vi "Main.vi"(7 "sweep rate, /min":dbl=0.2, 8 "sweep to:":dbl=-0.5, 9 "sweep":T6(radio)=enum."time_sweep") -> ()   [LabVIEW 2017] (continued)
            n4932 = property on="Continuous Sweep" class="Bool (strict)"("DisabledEnum"=w6382) -> ()  [unwired: 2 in, 2 out]
            n4933 = property on="Step and Hyerloop Setups" class="TabCtl (strict)"() -> ("Pages"=w6368:refnum<vi>[])  [unwired: 2 in, 2 out]
            n4934 = property on="Step and Hyerloop Setups" class="TabCtl (strict)"() -> ("Pages"=w6374:refnum<vi>[])  [unwired: 2 in, 2 out]
            n4935 = Index Array(array=w6377, index=2) -> (element=w6378:refnum<vi>)
            n4936 = Index Array(array=w6368, index=3) -> (element=w6367:refnum<vi>)
            n4937 = Index Array(array=w6374, index=1) -> (element=w6373:refnum<vi>)
            n4938 = property on="Continuous Sweep" class="Bool (strict)"("Value"=FALSE ("Continuous Sweep")) -> ()  [unwired: 2 in, 2 out]
            n4939 = property on="SuperHyper" class="Bool (strict)"("Value"=FALSE ("SuperHyper")) -> ()  [unwired: 2 in, 2 out]
            n4940 = property class="Page"(reference=w6378, "PageVis"=FALSE ("Page Visible")) -> ()  [unwired: 1 in, 2 out]
            n4941 = property on="MappingName" class="Str"("Visible"=TRUE) -> ()  [unwired: 2 in, 2 out]
            n4942 = property class="Page"(reference=w6367, "PageVis"=FALSE ("Page Visible")) -> ()  [unwired: 1 in, 2 out]
            n4943 = property class="Page"(reference=w6373, "PageVis"=TRUE ("Page Visible")) -> ()  [unwired: 1 in, 2 out]
            n4944 = property on="step" class="RadioBtnsControl (strict)"("DisabledEnum"=w6380) -> ()  [unwired: 2 in, 2 out]
            n4945 = property on="diagonal step" class="Bool (strict)"("DisabledEnum"=w6380) -> ()  [unwired: 2 in, 2 out]
            n4946 = property on="Step Offset" class="DigNum (strict)"("DisabledEnum"=w6380) -> ()  [unwired: 2 in, 2 out]
            n4947 = property on="Step Slope" class="DigNum (strict)"("DisabledEnum"=w6380) -> ()  [unwired: 2 in, 2 out]
            n4948 = property on="FieldRate(T/min)" class="DigNum (strict)"("DisabledEnum"=w6380) -> ()  [unwired: 2 in, 2 out]
            n4949 = property on="iPS _addr_step" class="VISAName"("DisabledEnum"=w6380) -> ()  [unwired: 2 in, 2 out]
            n4950 = property on="wait between sweeps(s)" class="DigNum (strict)"("DisabledEnum"=w6380) -> ()  [unwired: 2 in, 2 out]
            n4951 = property on="2336A_addr_step" class="VISAName"("DisabledEnum"=w6380) -> ()  [unwired: 2 in, 2 out]
            n4952 = property on="iTC_addr_step" class="VISAName"("DisabledEnum"=w6380) -> ()  [unwired: 2 in, 2 out]
            n4953 = property on="Start Mapping" class="Bool"("DisabledEnum"=w6380) -> ()  [unwired: 2 in, 2 out]
            n4954 = property on="2400_1_addr_step" class="DigNum (strict)"("DisabledEnum"=w6380) -> ()  [unwired: 2 in, 2 out]
            n4955 = property on="Tolerance_Step" class="DigNum (strict)"("DisabledEnum"=w6380) -> ()  [unwired: 2 in, 2 out]
            n4956 = property on="Wait Between Step(s)" class="DigNum (strict)"("DisabledEnum"=w6380) -> ()  [unwired: 2 in, 2 out]
            n4957 = property on="2400_2_addr_step" class="DigNum (strict)"("DisabledEnum"=w6380) -> ()  [unwired: 2 in, 2 out]
            n4958 = property on="HyperLoop" class="Bool (strict)"("DisabledEnum"=w6380) -> ()  [unwired: 2 in, 2 out]
          }
          frame False {
            w6393 = T12."Disabled and Grayed Out" ("Disabled")
            w6400 = T12."Enabled" ("Disabled")
            n4959 = property on="Ramp\n Down" class="Bool"("DisabledEnum"=w6400) -> ()  [unwired: 2 in, 2 out]
            n4960 = property on="iTC_addr_sweep" class="VISAName"("DisabledEnum"=w6400) -> ()  [unwired: 2 in, 2 out]
            n4961 = property on="sweep" class="RadioBtnsControl (strict)"("DisabledEnum"=w6400) -> ()  [unwired: 2 in, 2 out]
            n4962 = property on="2182A 1 addr" class="DigNum (strict)"("DisabledEnum"=w6400) -> ()  [unwired: 2 in, 2 out]
            n4963 = property on="2182A 2 addr" class="DigNum (strict)"("DisabledEnum"=w6400) -> ()  [unwired: 2 in, 2 out]
            n4964 = property on="2182A 3 addr" class="DigNum (strict)"("DisabledEnum"=w6400) -> ()  [unwired: 2 in, 2 out]
            n4965 = property on="2182A 4 addr" class="DigNum (strict)"("DisabledEnum"=w6400) -> ()  [unwired: 2 in, 2 out]
            n4966 = property on="2400 1 addr" class="DigNum (strict)"("DisabledEnum"=w6400) -> ()  [unwired: 2 in, 2 out]
            n4967 = property on="iPS_addr_sweep" class="VISAName"("DisabledEnum"=w6400) -> ()  [unwired: 2 in, 2 out]
            n4968 = property on="Sweep Down" class="Bool"("DisabledEnum"=w6400) -> ()  [unwired: 2 in, 2 out]
            n4969 = property on="SR830 2 addr" class="DigNum (strict)"("DisabledEnum"=w6400) -> ()  [unwired: 2 in, 2 out]
            n4970 = property on="SR830 3 addr" class="DigNum (strict)"("DisabledEnum"=w6400) -> ()  [unwired: 2 in, 2 out]
            n4971 = property on="2400 2 addr" class="DigNum (strict)"("DisabledEnum"=w6400) -> ()  [unwired: 2 in, 2 out]
            n4972 = property on="2400 3 addr" class="DigNum (strict)"("DisabledEnum"=w6400) -> ()  [unwired: 2 in, 2 out]
            n4973 = property on="2336A addr" class="VISAName"("DisabledEnum"=w6400) -> ()  [unwired: 2 in, 2 out]
            n4974 = property on="SR830 1 addr" class="DigNum (strict)"("DisabledEnum"=w6400) -> ()  [unwired: 2 in, 2 out]
            n4975 = property on="SR830 4 addr" class="DigNum (strict)"("DisabledEnum"=w6400) -> ()  [unwired: 2 in, 2 out]
            n4976 = property on="Ramp \nUp" class="Bool"("DisabledEnum"=w6400) -> ()  [unwired: 2 in, 2 out]
            n4977 = property on="Sweep Up" class="Bool"("DisabledEnum"=w6400) -> ()  [unwired: 2 in, 2 out]
            n4978 = property on="Step and Hyerloop Setups" class="TabCtl (strict)"() -> ("Pages"=w6388:refnum<vi>[])  [unwired: 2 in, 2 out]
            n4979 = property on="Step and Hyerloop Setups" class="TabCtl (strict)"() -> ("Pages"=w6387:refnum<vi>[])  [unwired: 2 in, 2 out]
            n4980 = property on="Tolerance_Sweep" class="DigNum (strict)"("DisabledEnum"=w6400) -> ()  [unwired: 2 in, 2 out]
            n4981 = property on="Continuous Sweep" class="Bool (strict)"("DisabledEnum"=w6400) -> ()  [unwired: 2 in, 2 out]
            n4982 = property on="Step and Hyerloop Setups" class="TabCtl (strict)"() -> ("Pages"=w6398:refnum<vi>[])  [unwired: 2 in, 2 out]
            n4983 = Index Array(array=w6388, index=2) -> (element=w6389:refnum<vi>)
            n4984 = Index Array(array=w6387, index=3) -> (element=w6386:refnum<vi>)
            n4985 = property on="MappingName" class="Str"("Visible"=FALSE) -> ()  [unwired: 2 in, 2 out]
            n4986 = Index Array(array=w6398, index=1) -> (element=w6397:refnum<vi>)
            n4987 = property class="Page"(reference=w6389, "PageVis"=FALSE ("Page Visible")) -> ()  [unwired: 1 in, 2 out]
            n4988 = property on="SuperHyper" class="Bool (strict)"("Value"=FALSE ("SuperHyper")) -> ()  [unwired: 2 in, 2 out]
            n4989 = property class="Page"(reference=w6386, "PageVis"=FALSE ("Page Visible")) -> ()  [unwired: 1 in, 2 out]
            n4990 = property on="HyperLoop" class="Bool (strict)"("Value"=FALSE ("HyperLoop")) -> ()  [unwired: 2 in, 2 out]
            n4991 = property class="Page"(reference=w6397, "PageVis"=FALSE ("Page Visible")) -> ()  [unwired: 1 in, 2 out]
            n4992 = property on="step" class="RadioBtnsControl (strict)"("DisabledEnum"=w6393) -> ()  [unwired: 2 in, 2 out]
            n4993 = property on="diagonal step" class="Bool (strict)"("DisabledEnum"=w6393) -> ()  [unwired: 2 in, 2 out]
            n4994 = property on="Step Offset" class="DigNum (strict)"("DisabledEnum"=w6393) -> ()  [unwired: 2 in, 2 out]
            n4995 = property on="Step Slope" class="DigNum (strict)"("DisabledEnum"=w6393) -> ()  [unwired: 2 in, 2 out]
            n4996 = property on="iPS _addr_step" class="VISAName"("DisabledEnum"=w6393) -> ()  [unwired: 2 in, 2 out]
            n4997 = property on="wait between sweeps(s)" class="DigNum (strict)"("DisabledEnum"=w6393) -> ()  [unwired: 2 in, 2 out]
            n4998 = property on="2336A_addr_step" class="VISAName"("DisabledEnum"=w6393) -> ()  [unwired: 2 in, 2 out]
            n4999 = property on="iTC_addr_step" class="VISAName"("DisabledEnum"=w6393) -> ()  [unwired: 2 in, 2 out]
            n5000 = property on="Start Mapping" class="Bool"("DisabledEnum"=w6393) -> ()  [unwired: 2 in, 2 out]
            n5001 = property on="2400_1_addr_step" class="DigNum (strict)"("DisabledEnum"=w6393) -> ()  [unwired: 2 in, 2 out]
            n5002 = property on="Wait Between Step(s)" class="DigNum (strict)"("DisabledEnum"=w6393) -> ()  [unwired: 2 in, 2 out]
            n5003 = property on="2400_2_addr_step" class="DigNum (strict)"("DisabledEnum"=w6393) -> ()  [unwired: 2 in, 2 out]
            n5004 = property on="FieldRate(T/min)" class="DigNum (strict)"("DisabledEnum"=w6393) -> ()  [unwired: 2 in, 2 out]
            n5005 = property on="Tolerance_Step" class="DigNum (strict)"("DisabledEnum"=w6393) -> ()  [unwired: 2 in, 2 out]
            n5006 = property on="HyperLoop" class="Bool (strict)"("DisabledEnum"=w6393) -> ()  [unwired: 2 in, 2 out]
          }
        }
      }
      event "Change Sweep Range": Value Change {
        n5007 = event-data() -> ()  [unwired: 1 in, 6 out]
        n5008 = property on="Change Sweep Range" class="Bool (strict)"() -> ("Value"=w6401:bool)  [unwired: 2 in, 2 out]
        n5009 = case shown="False" w6401 {
          frame False {
            w6402 = FALSE ("Visible")
            n5010 = property on="UpLimitValue" class="DigNum (strict)"("Visible"=w6402) -> ()  [unwired: 2 in, 2 out]
            n5011 = property on="DownLimitValue" class="DigNum (strict)"("Visible"=w6402) -> ()  [unwired: 2 in, 2 out]
            n5012 = property on="Generate" class="Bool"("Visible"=w6402) -> ()  [unwired: 2 in, 2 out]
            n5013 = property on="Offset_Up" class="DigNum (strict)"("Visible"=w6402) -> ()  [unwired: 2 in, 2 out]
            n5014 = property on="Down          Up" class="Tbl (strict)"("Visible"=w6402) -> ()  [unwired: 2 in, 2 out]
            n5015 = property on="Slope" class="DigNum (strict)"("Visible"=w6402) -> ()  [unwired: 2 in, 2 out]
            n5016 = property on="Offset_Down" class="DigNum (strict)"("Visible"=w6402) -> ()  [unwired: 2 in, 2 out]
          }
          frame True {
            w6403 = TRUE ("Visible")
            n5017 = property on="UpLimitValue" class="DigNum (strict)"("Visible"=w6403) -> ()  [unwired: 2 in, 2 out]
            n5018 = property on="Generate" class="Bool"("Visible"=w6403) -> ()  [unwired: 2 in, 2 out]
            n5019 = property on="DownLimitValue" class="DigNum (strict)"("Visible"=w6403) -> ()  [unwired: 2 in, 2 out]
            n5020 = property on="Offset_Up" class="DigNum (strict)"("Visible"=w6403) -> ()  [unwired: 2 in, 2 out]
            n5021 = property on="Down          Up" class="Tbl (strict)"("Visible"=w6403) -> ()  [unwired: 2 in, 2 out]
            n5022 = property on="Slope" class="DigNum (strict)"("Visible"=w6403) -> ()  [unwired: 2 in, 2 out]
            n5023 = property on="Offset_Down" class="DigNum (strict)"("Visible"=w6403) -> ()  [unwired: 2 in, 2 out]
          }
        }
      }
      event "Generate": Value Change {
        n5024 = event-data() -> ()  [unwired: 1 in, 6 out]
        n5025 = stacked-sequence {
          frame #0 {
            # "Initialize the background colours of cells"
            n5026 = property on="Down          Up" class="Tbl (strict)"("Active Cell"=cluster{"Row":i32, "Column":i32} {"Row"=-2, "Column"=-2}, "Cell BG Color"=u32 16448250 ("Active Cell:Cell Background Color")) -> ()  [unwired: 2 in, 2 out]
          }
          frame #1 {
            # "Fill the tables"
            n5027 = property on="Step values" class="Tbl (strict)"() -> ("Value"=w6413:string[][])  [unwired: 2 in, 2 out]
            n5028 = Index Array(array=w6413, index (col)=0 ("index (row)")) -> (element=w6410:string[])  [unwired: 1 in]
            n5029 = Array Size(array=w6410) -> (size(s)=w6412:i32)
            n5030 = for {
              N: w6412 -> [_]
              tunnel: [w6433] -> w6409 mode=indexing
              tunnel: [w6432] -> w6408 mode=indexing
              i -> [w6429]
              n5031 = property on="Step values" class="Tbl (strict)"() -> ("Value"=w6431:string[][])  [unwired: 2 in, 2 out]
              n5032 = property on="Slope" class="DigNum (strict)"() -> ("Value"=w6435:dbl)  [unwired: 2 in, 2 out]
              n5033 = Index Array(array=w6431, index (row)=w6429, index (col)=0 ("disabled index (col)")) -> (element=w6428:string)
              n5034 = Fract/Exp String To Number(string=w6428) -> (number=w6414:dbl)  [unwired: 3 in, 1 out]
              n5035 = property on="Offset_Up" class="DigNum (strict)"() -> ("Value"=w6434:dbl)  [unwired: 2 in, 2 out]
              n5036 = Multiply(x=w6414, y=w6435) -> (x*y=w6425:dbl)
              n5037 = property on="Offset_Down" class="DigNum (strict)"() -> ("Value"=w6426:dbl)  [unwired: 2 in, 2 out]
              n5038 = property on="UpLimitValue" class="DigNum (strict)"() -> ("Value"=w6420:dbl)  [unwired: 2 in, 2 out]
              n5039 = Add(x=w6425, y=w6434) -> (x+y=w6421:dbl)
              n5040 = Add(x=w6426, y=w6425) -> (x+y=w6424:dbl)
              n5041 = property on="DownLimitValue" class="DigNum (strict)"() -> ("Value"=w6423:dbl)  [unwired: 2 in, 2 out]
              n5042 = property on="Change Doule Sweep OffSet" class="Bool (strict)"() -> ("Value"=w6419:bool)  [unwired: 2 in, 2 out]
              n5043 = Less?(x=w6421, y=w6420) -> (x < y?=w6422:bool)
              n5044 = Greater?(x=w6424, y=w6423) -> (0:w6427:bool)
              n5045 = Select(t=w6421, s=w6422, f=w6420) -> (s? t:f=w6416:dbl)
              n5046 = Select(t=w6424, s=w6427, f=w6423) -> (s? t:f=w6417:dbl)
              n5047 = case shown="True" w6419 {
                tunnel: [w6437 w6449] -> w6418
                tunnel: w6417 -> [w6437 w6445]
                tunnel: [w6436 w6448] -> w6415
                tunnel: w6416 -> [w6436 w6441]
                tunnel: w6414 -> [_ w6453]
                frame False {
                }
                frame True {
                  n5048 = property on="Slope" class="DigNum (strict)"() -> ("Value"=w6446:dbl)  [unwired: 2 in, 2 out]
                  n5049 = property on="SlaveUpLimit" class="DigNum (strict)"() -> ("Value"=w6454:dbl)  [unwired: 2 in, 2 out]
                  n5050 = property on="SlaveDownLimit" class="DigNum (strict)"() -> ("Value"=w6455:dbl)  [unwired: 2 in, 2 out]
                  n5051 = Absolute Value(x=w6441) -> (abs(x)=w6440:dbl)
                  n5052 = Subtract(x=w6454, y=w6453) -> (x-y=w6451:dbl)
                  n5053 = Subtract(x=w6455, y=w6453) -> (x-y=w6452:dbl)
                  n5054 = Absolute Value(x=w6445) -> (abs(x)=w6444:dbl)
                  n5055 = Divide(x=w6452, y=w6446) -> (x/y=w6443:dbl)
                  n5056 = Divide(x=w6451, y=w6446) -> (x/y=w6438:dbl)
                  n5057 = Absolute Value(x=w6438) -> (abs(x)=w6439:dbl)
                  n5058 = Absolute Value(x=w6443) -> (abs(x)=w6442:dbl)
                  n5059 = Less?(x=w6442, y=w6444) -> (x < y?=w6450:bool)
                  n5060 = Less?(x=w6439, y=w6440) -> (x < y?=w6447:bool)
                  n5061 = Select(t=w6438, s=w6447, f=w6441) -> (s? t:f=w6448:dbl)
                  n5062 = Select(t=w6443, s=w6450, f=w6445) -> (s? t:f=w6449:dbl)
                }
              }
              n5063 = Number To Fractional String(number=w6415) -> (F-format string=w6432:string)  [unwired: 3 in]
              n5064 = Number To Fractional String(number=w6418) -> (F-format string=w6433:string)  [unwired: 3 in]
            }
            n5065 = Build Array(w6409, w6408) -> (w6407:string[][])
            n5066 = Transpose 2D Array(2D array=w6407) -> (transposed array=w6406:string[][])
            n5067 = property on="Down          Up" class="Tbl (strict)"("Value"=w6406) -> ()  [unwired: 2 in, 2 out]
          }
        }
      }
      event "HyperLoop": Value Change {
        n5068 = event-data() -> ()  [unwired: 1 in, 6 out]
        n5069 = property on="HyperLoop" class="Bool (strict)"() -> ("Value"=w6456:bool)  [unwired: 2 in, 2 out]
        n5070 = case shown="True" w6456 {
          frame False {
            n5071 = property on="Step and Hyerloop Setups" class="TabCtl (strict)"() -> ("Pages"=w6462:refnum<vi>[])  [unwired: 2 in, 2 out]
            n5072 = Index Array(array=w6462, index=3) -> (element=w6461:refnum<vi>)
            n5073 = property on="SuperHyper" class="Bool (strict)"("Value"=FALSE ("SuperHyper")) -> ()  [unwired: 2 in, 2 out]
            n5074 = property on="HyperLoop" class="Bool (strict)"("Value"=FALSE ("HyperLoop")) -> ()  [unwired: 2 in, 2 out]
            n5075 = property class="Page"(reference=w6461, "PageVis"=FALSE ("Page Visible")) -> ()  [unwired: 1 in, 2 out]
            n5076 = property on="Step and Hyerloop Setups" class="TabCtl (strict)"() -> ("Pages"=w6467:refnum<vi>[])  [unwired: 2 in, 2 out]
            n5077 = Index Array(array=w6467, index=2) -> (element=w6466:refnum<vi>)
            n5078 = property on="Start Mapping" class="Bool"("DisabledEnum"=T12."Enabled" ("Disabled")) -> ()  [unwired: 2 in, 2 out]
            n5079 = property class="Page"(reference=w6466, "PageVis"=FALSE ("Page Visible")) -> ()  [unwired: 1 in, 2 out]
          }
          frame True {
            n5080 = property on="Step and Hyerloop Setups" class="TabCtl (strict)"() -> ("Pages"=w6473:refnum<vi>[])  [unwired: 2 in, 2 out]
            n5081 = Index Array(array=w6473, index=2) -> (element=w6471:refnum<vi>)
            n5082 = property on="Start Mapping" class="Bool"("DisabledEnum"=T12."Disabled and Grayed Out" ("Disabled")) -> ()  [unwired: 2 in, 2 out]
            n5083 = property class="Page"(reference=w6471, "PageVis"=TRUE ("Page Visible")) -> ()  [unwired: 1 in, 2 out]
            n5084 = property on="SuperHyper" class="Bool (strict)"("Value"=FALSE ("SuperHyper")) -> ()  [unwired: 2 in, 2 out]
          }
        }
      }
      event "SuperHyper": Value Change {
        n5085 = event-data() -> ()  [unwired: 1 in, 6 out]
        n5086 = property on="SuperHyper" class="Bool (strict)"() -> ("Value"=w6474:bool)  [unwired: 2 in, 2 out]
        n5087 = case shown="True" w6474 {
          frame False {
            n5088 = property on="Step and Hyerloop Setups" class="TabCtl (strict)"() -> ("Pages"=w6479:refnum<vi>[])  [unwired: 2 in, 2 out]
            n5089 = Index Array(array=w6479, index=3) -> (element=w6478:refnum<vi>)
            n5090 = property on="Start HyperLoop" class="Bool"("DisabledEnum"=T12."Enabled" ("Disabled")) -> ()  [unwired: 2 in, 2 out]
            n5091 = property class="Page"(reference=w6478, "PageVis"=FALSE ("Page Visible")) -> ()  [unwired: 1 in, 2 out]
          }
          frame True {
            n5092 = property on="Step  Setups" class="TabCtl (strict)"() -> ("Pages"=w6484:refnum<vi>[])  [unwired: 2 in, 2 out]
            n5093 = Index Array(array=w6484, index=3) -> (element=w6482:refnum<vi>)
            n5094 = property class="Page"(reference=w6482, "PageVis"=TRUE ("Page Visible")) -> ()  [unwired: 1 in, 2 out]
            n5095 = property on="Start HyperLoop" class="Bool"("DisabledEnum"=T12."Disabled and Grayed Out" ("Disabled")) -> ()  [unwired: 2 in, 2 out]
          }
        }
      }
      event "Quit": Value Change {
        n5096 = event-data() -> ()  [unwired: 1 in, 6 out]
        n5097 = Flush Queue(queue=w6487) -> (queue out=w6486:refnum<queue>)  [unwired: 1 in, 2 out]
        n5098 = Enqueue Element(queue=w6486, element="Quit") -> ()  [unwired: 2 in, 3 out]
      }
      event "Populate step table?": Value Change {
        n5099 = event-data() -> ()  [unwired: 1 in, 6 out]
        n5100 = stacked-sequence {
          frame #0 {
            # "Initialize the background colours of cells"
            n5101 = property on="Step values" class="Tbl (strict)"("Active Cell"=cluster{"Row":i32, "Column":i32} {"Row"=-2, "Column"=-2}, "Cell BG Color"=u32 16448250 ("Active Cell:Cell Background Color")) -> ()  [unwired: 2 in, 2 out]
          }
          frame #1 {
            # "Fill the tables"
            n5102 = property on="to" class="DigNum (strict)"() -> ("Value"=w6492:dbl)  [unwired: 2 in, 2 out]
            n5103 = property on="step" class="DigNum (strict)"() -> ("Value"=w6491:dbl)  [unwired: 2 in, 2 out]
            n5104 = property on="from" class="DigNum (strict)"() -> ("Value"=w6493:dbl)  [unwired: 2 in, 2 out]
            n5105 = Subtract(x=w6493, y=w6492) -> (x-y=w6500:dbl)
            n5106 = Divide(x=w6500, y=w6491) -> (x/y=w6499:dbl)
            n5107 = Sign(1:w6500) -> (0:w6503:dbl)
            n5108 = Absolute Value(x=w6499) -> (abs(x)=w6498:dbl)
            n5109 = Negate(x=w6503) -> (-x=w6495:dbl)
            n5110 = Round Toward -Infinity(1:w6498) -> (0:w6497:dbl)
            n5111 = Increment(x=w6497) -> (x+1=w6496:dbl)
            n5112 = for {
              N: w6496 -> [_]
              tunnel: w6493 -> [w6509]
              tunnel: w6495 -> [w6510]
              tunnel: w6491 -> [w6512]
              tunnel: [w6506] -> w6501 mode=indexing
              i -> [w6504]
              n5113 = Multiply(x=w6512, y=w6504) -> (x*y=w6511:dbl)
              n5114 = Multiply(x=w6510, y=w6511) -> (x*y=w6508:dbl)
              n5115 = Add(x=w6509, y=w6508) -> (x+y=w6507:dbl)
              n5116 = Number To Fractional String(number=w6507, precision (6)=i16 6) -> (F-format string=w6506:string)  [unwired: 2 in]
            }
            n5117 = Build Array(w6501) -> (w6502:string[][])
            n5118 = Transpose 2D Array(2D array=w6502) -> (transposed array=w6494:string[][])
            n5119 = property on="Step values" class="Tbl (strict)"("Value"=w6494) -> ()  [unwired: 2 in, 2 out]
          }
          frame #2 {
            # "Calculate the measurement time and estimate the finished time"
            n5120 = property on="upper limit" class="DigNum (strict)"() -> ("Value"=w6544:dbl)  [unwired: 2 in, 2 out]
            n5121 = property on="lower limit" class="DigNum (strict)"() -> ("Value"=w6545:dbl)  [unwired: 2 in, 2 out]
            n5122 = Subtract(x=w6545, y=w6544) -> (x-y=w6543:dbl)
            n5123 = property on="Down Rate" class="DigNum (strict)"() -> ("Value"=w6540:dbl)  [unwired: 2 in, 2 out]
            n5124 = property on="Up Rate" class="DigNum (strict)"() -> ("Value"=w6542:dbl)  [unwired: 2 in, 2 out]
            n5125 = Absolute Value(x=w6543) -> (abs(x)=w6541:dbl)
            n5126 = property on="step" class="RadioBtnsControl (strict)"() -> ("Value"=w6520:T8)  [unwired: 2 in, 2 out]
            n5127 = Divide(x=w6541, y=w6542) -> (x/y=w6539:dbl)
            n5128 = Divide(x=w6541, y=w6540) -> (x/y=w6538:dbl)
            n5129 = case shown="\"iPS_step\"" w6520 {
              tunnel: [w6546 0.0] -> w6516
              frame "iPS_step" {
                n5130 = property on="step" class="DigNum (strict)"() -> ("Value"=w6550:dbl)  [unwired: 2 in, 2 out]
                n5131 = property on="FieldRate(T/min)" class="DigNum (strict)"() -> ("Value"=w6549:dbl)  [unwired: 2 in, 2 out]
                n5132 = Divide(x=w6550, y=w6549) -> (x/y=w6548:dbl)
                n5133 = Multiply(x=w6548, y=60.0) -> (x*y=w6546:dbl)
              }
              frame "V2400_1_Step".."iTC_step", Default {
              }
            }
            n5134 = property on="Wait Between Step(s)" class="DigNum (strict)"() -> ("Value"=w6535:i32)  [unwired: 2 in, 2 out]
            n5135 = Add(x=w6539, y=w6538) -> (x+y=w6537:dbl)
            n5136 = Multiply(x=w6537, y=60.0) -> (x*y=w6536:dbl)
            n5137 = property on="Step values" class="Tbl (strict)"() -> ("Value"=w6530:string[][])  [unwired: 2 in, 2 out]
            n5138 = property on="wait between sweeps(s)" class="DigNum (strict)"() -> ("Value"=w6533:u32)  [unwired: 2 in, 2 out]
            n5139 = Add(x=w6536, y=w6535) -> (x+y=w6534:dbl)
            n5140 = Array Size(array=w6530) -> (size(s)=w6529:i32[])
            n5141 = Index Array(array=w6529, index=0) -> (element=w6515:i32)
            n5142 = Add(x=w6534, y=w6533) -> (x+y=w6519:dbl)
            n5143 = Multiply(x=w6515, y=w6519) -> (x*y=w6517:dbl)
            n5144 = Decrement(x=w6515) -> (x-1=w6514:i32)
            n5145 = Multiply(x=w6514, y=w6516) -> (x*y=w6513:dbl)
            n5146 = Add(x=w6517, y=w6513) -> (x+y=w6518:dbl)
            n5147 = Get Date/Time In Seconds() -> (seconds since 1Jan1904=w6532:timestamp)
            n5148 = Add(x=w6518, y=w6532) -> (x+y=w6528:timestamp)
            n5149 = Quotient & Remainder(x=w6518, y=3600.0) -> (x-y*floor(x/y)=w6531:dbl, floor(x/y)=w6527:dbl)
            n5150 = Quotient & Remainder(x=w6531, y=60.0) -> (x-y*floor(x/y)=w6525:dbl, floor(x/y)=w6526:dbl)
            n5151 = property on="SS:" class="DigNum (strict)"("Value"=w6525) -> ()  [unwired: 2 in, 2 out]
            n5152 = property on="MM:" class="DigNum (strict)"("Value"=w6526) -> ()  [unwired: 2 in, 2 out]
            n5153 = property on="HH:" class="DigNum (strict)"("Value"=w6527) -> ()  [unwired: 2 in, 2 out]
            n5154 = property on="Finish Time" class="AbsTime (strict)"("Value"=w6528) -> ()  [unwired: 2 in, 2 out]
          }
        }
      }
      event "Hidden_HyperLoop_Swap": Value Change {
        n5155 = event-data() -> ()  [unwired: 1 in, 6 out]
        n5156 = stacked-sequence {
          frame #0 {
            # "Initialize the background colours of cells"
            n5157 = property on="Step values" class="Tbl (strict)"("Active Cell"=cluster{"Row":i32, "Column":i32} {"Row"=-2, "Column"=-2}, "Cell BG Color"=u32 16448250 ("Active Cell:Cell Background Color")) -> ()  [unwired: 2 in, 2 out]
          }
          frame #1 {
            # "Fill the tables"
            n5158 = property on="Step values" class="Tbl (strict)"() -> ("Value"=w6559:string[][])  [unwired: 2 in, 2 out]
            n5159 = Index Array(array=w6559, index (col)=0 ("disabled index (col)")) -> (element=w6557:string[])  [unwired: 1 in]
            n5160 = Reverse 1D Array(array=w6557) -> (reversed array=w6556:string[])
            n5161 = Build Array(w6556) -> (w6555:string[][])
            n5162 = Transpose 2D Array(2D array=w6555) -> (transposed array=w6554:string[][])
            n5163 = property on="Step values" class="Tbl (strict)"("Value"=w6554) -> ()  [unwired: 2 in, 2 out]
          }
          frame #2 {
            # "Calculate the measurement time and estimate the finished time"
            n5164 = property on="upper limit" class="DigNum (strict)"() -> ("Value"=w6591:dbl)  [unwired: 2 in, 2 out]
            n5165 = property on="lower limit" class="DigNum (strict)"() -> ("Value"=w6592:dbl)  [unwired: 2 in, 2 out]
            n5166 = Subtract(x=w6592, y=w6591) -> (x-y=w6590:dbl)
            n5167 = property on="Down Rate" class="DigNum (strict)"() -> ("Value"=w6587:dbl)  [unwired: 2 in, 2 out]
            n5168 = property on="Up Rate" class="DigNum (strict)"() -> ("Value"=w6589:dbl)  [unwired: 2 in, 2 out]
            n5169 = Absolute Value(x=w6590) -> (abs(x)=w6588:dbl)
            n5170 = property on="step" class="RadioBtnsControl (strict)"() -> ("Value"=w6567:T8)  [unwired: 2 in, 2 out]
            n5171 = Divide(x=w6588, y=w6589) -> (x/y=w6586:dbl)
            n5172 = Divide(x=w6588, y=w6587) -> (x/y=w6585:dbl)
            n5173 = case shown="\"iPS_step\"" w6567 {
              tunnel: [w6593 0.0] -> w6563
              frame "iPS_step" {
                n5174 = property on="step" class="DigNum (strict)"() -> ("Value"=w6597:dbl)  [unwired: 2 in, 2 out]
                n5175 = property on="FieldRate(T/min)" class="DigNum (strict)"() -> ("Value"=w6596:dbl)  [unwired: 2 in, 2 out]
                n5176 = Divide(x=w6597, y=w6596) -> (x/y=w6595:dbl)
                n5177 = Multiply(x=w6595, y=60.0) -> (x*y=w6593:dbl)
              }
              frame "V2400_1_Step".."iTC_step", Default {
              }
            }
            n5178 = property on="Wait Between Step(s)" class="DigNum (strict)"() -> ("Value"=w6582:i32)  [unwired: 2 in, 2 out]
            n5179 = Add(x=w6586, y=w6585) -> (x+y=w6584:dbl)
            n5180 = Multiply(x=w6584, y=60.0) -> (x*y=w6583:dbl)
            n5181 = property on="Step values" class="Tbl (strict)"() -> ("Value"=w6577:string[][])  [unwired: 2 in, 2 out]
            n5182 = property on="wait between sweeps(s)" class="DigNum (strict)"() -> ("Value"=w6580:u32)  [unwired: 2 in, 2 out]
            n5183 = Add(x=w6583, y=w6582) -> (x+y=w6581:dbl)
            n5184 = Array Size(array=w6577) -> (size(s)=w6576:i32[])
            n5185 = Index Array(array=w6576, index=0) -> (element=w6562:i32)
            n5186 = Add(x=w6581, y=w6580) -> (x+y=w6566:dbl)
            n5187 = Multiply(x=w6562, y=w6566) -> (x*y=w6564:dbl)
            n5188 = Decrement(x=w6562) -> (x-1=w6561:i32)
            n5189 = Multiply(x=w6561, y=w6563) -> (x*y=w6560:dbl)
            n5190 = Add(x=w6564, y=w6560) -> (x+y=w6565:dbl)
            n5191 = Get Date/Time In Seconds() -> (seconds since 1Jan1904=w6579:timestamp)
            n5192 = Add(x=w6565, y=w6579) -> (x+y=w6575:timestamp)
            n5193 = Quotient & Remainder(x=w6565, y=3600.0) -> (x-y*floor(x/y)=w6578:dbl, floor(x/y)=w6574:dbl)
            n5194 = Quotient & Remainder(x=w6578, y=60.0) -> (x-y*floor(x/y)=w6572:dbl, floor(x/y)=w6573:dbl)
            n5195 = property on="SS:" class="DigNum (strict)"("Value"=w6572) -> ()  [unwired: 2 in, 2 out]
            n5196 = property on="MM:" class="DigNum (strict)"("Value"=w6573) -> ()  [unwired: 2 in, 2 out]
            n5197 = property on="HH:" class="DigNum (strict)"("Value"=w6574) -> ()  [unwired: 2 in, 2 out]
            n5198 = property on="Finish Time" class="AbsTime (strict)"("Value"=w6575) -> ()  [unwired: 2 in, 2 out]
          }
        }
      }
      event "Populate HyperLoop table?": Value Change {
        n5199 = event-data() -> ()  [unwired: 1 in, 6 out]
        n5200 = stacked-sequence {
          frame #0 {
            n5201 = property on="HyperLoop Steps" class="Tbl (strict)"("Active Cell"=cluster{"Row":i32, "Column":i32} {"Row"=-2, "Column"=-2}, "Cell BG Color"=u32 16448250 ("Active Cell:Cell Background Color")) -> ()  [unwired: 2 in, 2 out]
          }
          frame #1 {
            n5202 = property on="to" class="DigNum (strict)"() -> ("Value"=w6603:dbl)  [unwired: 2 in, 2 out]
            n5203 = property on="step" class="DigNum (strict)"() -> ("Value"=w6602:dbl)  [unwired: 2 in, 2 out]
            n5204 = property on="from" class="DigNum (strict)"() -> ("Value"=w6604:dbl)  [unwired: 2 in, 2 out]
            n5205 = Subtract(x=w6604, y=w6603) -> (x-y=w6610:dbl)
            n5206 = Divide(x=w6610, y=w6602) -> (x/y=w6609:dbl)
            n5207 = Sign(1:w6610) -> (0:w6613:dbl)
            n5208 = Absolute Value(x=w6609) -> (abs(x)=w6608:dbl)
            n5209 = Negate(x=w6613) -> (-x=w6605:dbl)
            n5210 = Round Toward -Infinity(1:w6608) -> (0:w6607:dbl)
            n5211 = Increment(x=w6607) -> (x+1=w6606:dbl)
            n5212 = for {
              N: w6606 -> [_]
              tunnel: w6604 -> [w6619]
              tunnel: w6605 -> [w6620]
              tunnel: w6602 -> [w6622]
              tunnel: [w6616] -> w6611 mode=indexing
              i -> [w6614]
              n5213 = Multiply(x=w6622, y=w6614) -> (x*y=w6621:dbl)
              n5214 = Multiply(x=w6620, y=w6621) -> (x*y=w6618:dbl)
              n5215 = Add(x=w6619, y=w6618) -> (x+y=w6617:dbl)
              n5216 = Number To Fractional String(number=w6617, precision (6)=i16 6) -> (F-format string=w6616:string)  [unwired: 2 in]
            }
            n5217 = Build Array(w6611) -> (w6612:string[][])
            n5218 = Transpose 2D Array(2D array=w6612) -> (transposed array=w6601:string[][])
            n5219 = property on="HyperLoop Steps" class="Tbl (strict)"("Value"=w6601) -> ()  [unwired: 2 in, 2 out]
          }
          frame #2 {
            n5220 = property on="upper limit" class="DigNum (strict)"() -> ("Value"=w6657:dbl)  [unwired: 2 in, 2 out]
            n5221 = property on="lower limit" class="DigNum (strict)"() -> ("Value"=w6658:dbl)  [unwired: 2 in, 2 out]
            n5222 = Subtract(x=w6658, y=w6657) -> (x-y=w6656:dbl)
            n5223 = property on="Down Rate" class="DigNum (strict)"() -> ("Value"=w6653:dbl)  [unwired: 2 in, 2 out]
            n5224 = property on="Up Rate" class="DigNum (strict)"() -> ("Value"=w6655:dbl)  [unwired: 2 in, 2 out]
            n5225 = Absolute Value(x=w6656) -> (abs(x)=w6654:dbl)
            n5226 = property on="step" class="RadioBtnsControl (strict)"() -> ("Value"=w6634:T8)  [unwired: 2 in, 2 out]
            n5227 = Divide(x=w6654, y=w6655) -> (x/y=w6652:dbl)
            n5228 = Divide(x=w6654, y=w6653) -> (x/y=w6651:dbl)
            n5229 = case shown="\"V2400_1_Step\"..\"iTC_step\", Default" w6634 {
              tunnel: [w6659 0.0] -> w6633
              frame "iPS_step" {
                n5230 = property on="step" class="DigNum (strict)"() -> ("Value"=w6663:dbl)  [unwired: 2 in, 2 out]
                n5231 = property on="FieldRate(T/min)" class="DigNum (strict)"() -> ("Value"=w6662:dbl)  [unwired: 2 in, 2 out]
                n5232 = Divide(x=w6663, y=w6662) -> (x/y=w6661:dbl)
                n5233 = Multiply(x=w6661, y=60.0) -> (x*y=w6659:dbl)
              }
              frame "V2400_1_Step".."iTC_step", Default {
              }
            }
            n5234 = property on="Wait Between Step(s)" class="DigNum (strict)"() -> ("Value"=w6648:i32)  [unwired: 2 in, 2 out]
            n5235 = Add(x=w6652, y=w6651) -> (x+y=w6650:dbl)
            n5236 = Multiply(x=w6650, y=60.0) -> (x*y=w6649:dbl)
            n5237 = property on="HyperLoop Steps" class="Tbl (strict)"() -> ("Value"=w6629:string[][])  [unwired: 2 in, 2 out]
            n5238 = property on="wait between sweeps(s)" class="DigNum (strict)"() -> ("Value"=w6646:u32)  [unwired: 2 in, 2 out]
            n5239 = Add(x=w6649, y=w6648) -> (x+y=w6647:dbl)
            n5240 = property on="Step values" class="Tbl (strict)"() -> ("Value"=w6643:string[][])  [unwired: 2 in, 2 out]
            n5241 = Array Size(array=w6629) -> (size(s)=w6631:i32[])
            n5242 = Array Size(array=w6643) -> (size(s)=w6642:i32[])
            n5243 = Add(x=w6647, y=w6646) -> (x+y=w6636:dbl)
            n5244 = Index Array(array=w6631, index=0) -> (element=w6632:i32)
            n5245 = Index Array(array=w6642, index=0) -> (element=w6641:i32)
            n5246 = Add(x=w6636, y=w6633) -> (x+y=w6635:dbl)
            n5247 = Multiply(x=w6641, y=w6635) -> (x*y=w6628:dbl)
            n5248 = Multiply(x=w6632, y=w6628) -> (x*y=w6627:dbl)
            n5249 = Get Date/Time In Seconds() -> (seconds since 1Jan1904=w6645:timestamp)
            n5250 = Add(x=w6627, y=w6645) -> (x+y=w6623:timestamp)
            n5251 = Quotient & Remainder(x=w6627, y=3600.0) -> (x-y*floor(x/y)=w6644:dbl, floor(x/y)=w6624:dbl)
            n5252 = Quotient & Remainder(x=w6644, y=60.0) -> (x-y*floor(x/y)=w6626:dbl, floor(x/y)=w6625:dbl)
            n5253 = property on="Finish Time 2" class="AbsTime (strict)"("Value"=w6623) -> ()  [unwired: 2 in, 2 out]
            n5254 = property on="HH:" class="DigNum (strict)"("Value"=w6624) -> ()  [unwired: 2 in, 2 out]
            n5255 = property on="MM:" class="DigNum (strict)"("Value"=w6625) -> ()  [unwired: 2 in, 2 out]
            n5256 = property on="SS:" class="DigNum (strict)"("Value"=w6626) -> ()  [unwired: 2 in, 2 out]
          }
        }
      }
      event "Populate SuperHyper table?": Value Change {
        n5257 = event-data() -> ()  [unwired: 1 in, 6 out]
        n5258 = stacked-sequence {
          frame #0 {
            n5259 = property on="SuperHyper Steps" class="Tbl (strict)"("Active Cell"=cluster{"Row":i32, "Column":i32} {"Row"=-2, "Column"=-2}, "Cell BG Color"=u32 16448250 ("Active Cell:Cell Background Color")) -> ()  [unwired: 2 in, 2 out]
          }
          frame #1 {
            n5260 = property on="to" class="DigNum (strict)"() -> ("Value"=w6669:dbl)  [unwired: 2 in, 2 out]
            n5261 = property on="from" class="DigNum (strict)"() -> ("Value"=w6670:dbl)  [unwired: 2 in, 2 out]
            n5262 = property on="step" class="DigNum (strict)"() -> ("Value"=w6668:dbl)  [unwired: 2 in, 2 out]
            n5263 = Subtract(x=w6670, y=w6669) -> (x-y=w6676:dbl)
            n5264 = Divide(x=w6676, y=w6668) -> (x/y=w6675:dbl)
            n5265 = Sign(1:w6676) -> (0:w6679:dbl)
            n5266 = Absolute Value(x=w6675) -> (abs(x)=w6674:dbl)
            n5267 = Negate(x=w6679) -> (-x=w6671:dbl)
            n5268 = Round Toward -Infinity(1:w6674) -> (0:w6673:dbl)
            n5269 = Increment(x=w6673) -> (x+1=w6672:dbl)
            n5270 = for {
              N: w6672 -> [_]
              tunnel: w6670 -> [w6685]
              tunnel: w6671 -> [w6686]
              tunnel: w6668 -> [w6688]
              tunnel: [w6682] -> w6677 mode=indexing
              i -> [w6680]
              n5271 = Multiply(x=w6688, y=w6680) -> (x*y=w6687:dbl)
              n5272 = Multiply(x=w6686, y=w6687) -> (x*y=w6684:dbl)
              n5273 = Add(x=w6685, y=w6684) -> (x+y=w6683:dbl)
              n5274 = Number To Fractional String(number=w6683, precision (6)=i16 6) -> (F-format string=w6682:string)  [unwired: 2 in]
            }
            n5275 = Build Array(w6677) -> (w6678:string[][])
            n5276 = Transpose 2D Array(2D array=w6678) -> (transposed array=w6667:string[][])
            n5277 = property on="SuperHyper Steps" class="Tbl (strict)"("Value"=w6667) -> ()  [unwired: 2 in, 2 out]
          }
          frame #2 {
            n5278 = property on="upper limit" class="DigNum (strict)"() -> ("Value"=w6728:dbl)  [unwired: 2 in, 2 out]
            n5279 = property on="lower limit" class="DigNum (strict)"() -> ("Value"=w6729:dbl)  [unwired: 2 in, 2 out]
            n5280 = Subtract(x=w6729, y=w6728) -> (x-y=w6727:dbl)
            n5281 = property on="Down Rate" class="DigNum (strict)"() -> ("Value"=w6724:dbl)  [unwired: 2 in, 2 out]
            n5282 = property on="Up Rate" class="DigNum (strict)"() -> ("Value"=w6726:dbl)  [unwired: 2 in, 2 out]
            n5283 = Absolute Value(x=w6727) -> (abs(x)=w6725:dbl)
            n5284 = property on="step" class="RadioBtnsControl (strict)"() -> ("Value"=w6705:T8)  [unwired: 2 in, 2 out]
            n5285 = Divide(x=w6725, y=w6726) -> (x/y=w6723:dbl)
            n5286 = Divide(x=w6725, y=w6724) -> (x/y=w6722:dbl)
            n5287 = case shown="\"iPS_step\"" w6705 {
              tunnel: [w6730 0.0] -> w6704
              frame "iPS_step" {
                n5288 = property on="step" class="DigNum (strict)"() -> ("Value"=w6734:dbl)  [unwired: 2 in, 2 out]
                n5289 = property on="FieldRate(T/min)" class="DigNum (strict)"() -> ("Value"=w6733:dbl)  [unwired: 2 in, 2 out]
                n5290 = Divide(x=w6734, y=w6733) -> (x/y=w6732:dbl)
                n5291 = Multiply(x=w6732, y=60.0) -> (x*y=w6730:dbl)
              }
              frame "V2400_1_Step".."iTC_step", Default {
              }
            }
            n5292 = property on="Wait Between Step(s)" class="DigNum (strict)"() -> ("Value"=w6719:i32)  [unwired: 2 in, 2 out]
            n5293 = Add(x=w6723, y=w6722) -> (x+y=w6721:dbl)
            n5294 = Multiply(x=w6721, y=60.0) -> (x*y=w6720:dbl)
            n5295 = property on="SuperHyper Steps" class="Tbl (strict)"() -> ("Value"=w6696:string[][])  [unwired: 2 in, 2 out]
            n5296 = property on="HyperLoop Steps" class="Tbl (strict)"() -> ("Value"=w6700:string[][])  [unwired: 2 in, 2 out]
            n5297 = property on="wait between sweeps(s)" class="DigNum (strict)"() -> ("Value"=w6717:u32)  [unwired: 2 in, 2 out]
            n5298 = Add(x=w6720, y=w6719) -> (x+y=w6718:dbl)
            n5299 = property on="Step values" class="Tbl (strict)"() -> ("Value"=w6714:string[][])  [unwired: 2 in, 2 out]
            n5300 = Array Size(array=w6700) -> (size(s)=w6702:i32[])
            n5301 = Array Size(array=w6696) -> (size(s)=w6697:i32[])
            n5302 = Array Size(array=w6714) -> (size(s)=w6713:i32[])
            n5303 = Add(x=w6718, y=w6717) -> (x+y=w6707:dbl)
            n5304 = Index Array(array=w6702, index=0) -> (element=w6703:i32)
            n5305 = Index Array(array=w6697, index=0) -> (element=w6695:i32)
            n5306 = Index Array(array=w6713, index=0) -> (element=w6712:i32)
            n5307 = Add(x=w6707, y=w6704) -> (x+y=w6706:dbl)
            n5308 = Multiply(x=w6712, y=w6706) -> (x*y=w6699:dbl)
            n5309 = Multiply(x=w6703, y=w6699) -> (x*y=w6694:dbl)
            n5310 = Multiply(x=w6695, y=w6694) -> (x*y=w6693:dbl)
            n5311 = Get Date/Time In Seconds() -> (seconds since 1Jan1904=w6716:timestamp)
            n5312 = Add(x=w6693, y=w6716) -> (x+y=w6692:timestamp)
            n5313 = Quotient & Remainder(x=w6693, y=3600.0) -> (x-y*floor(x/y)=w6715:dbl, floor(x/y)=w6691:dbl)
            n5314 = Quotient & Remainder(x=w6715, y=60.0) -> (x-y*floor(x/y)=w6689:dbl, floor(x/y)=w6690:dbl)
            n5315 = property on="HH:" class="DigNum (strict)"("Value"=w6691) -> ()  [unwired: 2 in, 2 out]
            n5316 = property on="Finish Time Super" class="AbsTime (strict)"("Value"=w6692) -> ()  [unwired: 2 in, 2 out]
            n5317 = property on="MM:" class="DigNum (strict)"("Value"=w6690) -> ()  [unwired: 2 in, 2 out]
            n5318 = property on="SS:" class="DigNum (strict)"("Value"=w6689) -> ()  [unwired: 2 in, 2 out]
          }
        }
      }
      event "EstimateTime Hyper": Value Change {
        n5319 = event-data() -> ()  [unwired: 1 in, 6 out]
        n5320 = property on="upper limit" class="DigNum (strict)"() -> ("Value"=w6770:dbl)  [unwired: 2 in, 2 out]
        n5321 = property on="lower limit" class="DigNum (strict)"() -> ("Value"=w6771:dbl)  [unwired: 2 in, 2 out]
        n5322 = Subtract(x=w6771, y=w6770) -> (x-y=w6769:dbl)
        n5323 = property on="Down Rate" class="DigNum (strict)"() -> ("Value"=w6766:dbl)  [unwired: 2 in, 2 out]
        n5324 = property on="Up Rate" class="DigNum (strict)"() -> ("Value"=w6768:dbl)  [unwired: 2 in, 2 out]
        n5325 = Absolute Value(x=w6769) -> (abs(x)=w6767:dbl)
        n5326 = property on="step" class="RadioBtnsControl (strict)"() -> ("Value"=w6747:T8)  [unwired: 2 in, 2 out]
        n5327 = Divide(x=w6767, y=w6768) -> (x/y=w6765:dbl)
        n5328 = Divide(x=w6767, y=w6766) -> (x/y=w6764:dbl)
        n5329 = case shown="\"iPS_step\"" w6747 {
          tunnel: [w6772 0.0] -> w6746
          frame "iPS_step" {
            n5330 = property on="step" class="DigNum (strict)"() -> ("Value"=w6776:dbl)  [unwired: 2 in, 2 out]
            n5331 = property on="FieldRate(T/min)" class="DigNum (strict)"() -> ("Value"=w6775:dbl)  [unwired: 2 in, 2 out]
            n5332 = Divide(x=w6776, y=w6775) -> (x/y=w6774:dbl)
            n5333 = Multiply(x=w6774, y=60.0) -> (x*y=w6772:dbl)
          }
          frame "V2400_1_Step".."iTC_step", Default {
          }
        }
        n5334 = property on="Wait Between Step(s)" class="DigNum (strict)"() -> ("Value"=w6761:i32)  [unwired: 2 in, 2 out]
        n5335 = Add(x=w6765, y=w6764) -> (x+y=w6763:dbl)
        n5336 = Multiply(x=w6763, y=60.0) -> (x*y=w6762:dbl)
        n5337 = property on="HyperLoop Steps" class="Tbl (strict)"() -> ("Value"=w6742:string[][])  [unwired: 2 in, 2 out]
        n5338 = property on="wait between sweeps(s)" class="DigNum (strict)"() -> ("Value"=w6759:u32)  [unwired: 2 in, 2 out]
        n5339 = Add(x=w6762, y=w6761) -> (x+y=w6760:dbl)
        n5340 = property on="Step values" class="Tbl (strict)"() -> ("Value"=w6756:string[][])  [unwired: 2 in, 2 out]
        n5341 = Array Size(array=w6742) -> (size(s)=w6744:i32[])
        n5342 = Array Size(array=w6756) -> (size(s)=w6755:i32[])
        n5343 = Add(x=w6760, y=w6759) -> (x+y=w6749:dbl)
        n5344 = Index Array(array=w6744, index=0) -> (element=w6745:i32)
        n5345 = Index Array(array=w6755, index=0) -> (element=w6754:i32)
        n5346 = Add(x=w6749, y=w6746) -> (x+y=w6748:dbl)
        n5347 = Multiply(x=w6754, y=w6748) -> (x*y=w6741:dbl)
        n5348 = Multiply(x=w6745, y=w6741) -> (x*y=w6740:dbl)
        n5349 = Get Date/Time In Seconds() -> (seconds since 1Jan1904=w6758:timestamp)
        n5350 = Add(x=w6740, y=w6758) -> (x+y=w6736:timestamp)
        n5351 = Quotient & Remainder(x=w6740, y=3600.0) -> (x-y*floor(x/y)=w6757:dbl, floor(x/y)=w6737:dbl)
        n5352 = Quotient & Remainder(x=w6757, y=60.0) -> (x-y*floor(x/y)=w6739:dbl, floor(x/y)=w6738:dbl)
        n5353 = property on="Finish Time 2" class="AbsTime (strict)"("Value"=w6736) -> ()  [unwired: 2 in, 2 out]
        n5354 = property on="HH:" class="DigNum (strict)"("Value"=w6737) -> ()  [unwired: 2 in, 2 out]
        n5355 = property on="MM:" class="DigNum (strict)"("Value"=w6738) -> ()  [unwired: 2 in, 2 out]
        n5356 = property on="SS:" class="DigNum (strict)"("Value"=w6739) -> ()  [unwired: 2 in, 2 out]
      }
      event "EstimateTime": Value Change {
        n5357 = event-data() -> ()  [unwired: 1 in, 6 out]
        n5358 = property on="upper limit" class="DigNum (strict)"() -> ("Value"=w6809:dbl)  [unwired: 2 in, 2 out]
        n5359 = property on="lower limit" class="DigNum (strict)"() -> ("Value"=w6810:dbl)  [unwired: 2 in, 2 out]
        n5360 = Subtract(x=w6810, y=w6809) -> (x-y=w6808:dbl)
        n5361 = property on="Down Rate" class="DigNum (strict)"() -> ("Value"=w6805:dbl)  [unwired: 2 in, 2 out]
        n5362 = property on="Up Rate" class="DigNum (strict)"() -> ("Value"=w6807:dbl)  [unwired: 2 in, 2 out]
        n5363 = Absolute Value(x=w6808) -> (abs(x)=w6806:dbl)
        n5364 = property on="step" class="RadioBtnsControl (strict)"() -> ("Value"=w6785:T8)  [unwired: 2 in, 2 out]
        n5365 = Divide(x=w6806, y=w6807) -> (x/y=w6804:dbl)
        n5366 = Divide(x=w6806, y=w6805) -> (x/y=w6803:dbl)
        n5367 = case shown="\"iPS_step\"" w6785 {
          tunnel: [w6811 0.0] -> w6783
          frame "iPS_step" {
            n5368 = property on="step" class="DigNum (strict)"() -> ("Value"=w6815:dbl)  [unwired: 2 in, 2 out]
            n5369 = property on="FieldRate(T/min)" class="DigNum (strict)"() -> ("Value"=w6814:dbl)  [unwired: 2 in, 2 out]
            n5370 = Divide(x=w6815, y=w6814) -> (x/y=w6813:dbl)
            n5371 = Multiply(x=w6813, y=60.0) -> (x*y=w6811:dbl)
          }
          frame "V2400_1_Step".."iTC_step", Default {
          }
        }
        n5372 = property on="Wait Between Step(s)" class="DigNum (strict)"() -> ("Value"=w6800:i32)  [unwired: 2 in, 2 out]
        n5373 = Add(x=w6804, y=w6803) -> (x+y=w6802:dbl)
        n5374 = Multiply(x=w6802, y=60.0) -> (x*y=w6801:dbl)
        n5375 = property on="Step values" class="Tbl (strict)"() -> ("Value"=w6791:string[][])  [unwired: 2 in, 2 out]
        n5376 = property on="wait between sweeps(s)" class="DigNum (strict)"() -> ("Value"=w6798:u32)  [unwired: 2 in, 2 out]
        n5377 = Add(x=w6801, y=w6800) -> (x+y=w6799:dbl)
        n5378 = Array Size(array=w6791) -> (size(s)=w6790:i32[])
        n5379 = property on="Table Index" class="DigNum (strict)"() -> ("Value"=w6779:dbl)  [unwired: 2 in, 2 out]
        n5380 = Index Array(array=w6790, index=0) -> (element=w6780:i32)
        n5381 = Add(x=w6799, y=w6798) -> (x+y=w6784:dbl)
        n5382 = Subtract(x=w6780, y=w6779) -> (x-y=w6778:dbl)
        n5383 = Add(x=w6784, y=w6783) -> (x+y=w6782:dbl)
        n5384 = Get Date/Time In Seconds() -> (seconds since 1Jan1904=w6797:timestamp)
        n5385 = Multiply(x=w6778, y=w6782) -> (x*y=w6796:dbl)
        n5386 = Add(x=w6796, y=w6797) -> (x+y=w6789:timestamp)
        n5387 = Quotient & Remainder(x=w6796, y=3600.0) -> (x-y*floor(x/y)=w6795:dbl, floor(x/y)=w6788:dbl)
        n5388 = Quotient & Remainder(x=w6795, y=60.0) -> (x-y*floor(x/y)=w6786:dbl, floor(x/y)=w6787:dbl)
        n5389 = property on="SS:" class="DigNum (strict)"("Value"=w6786) -> ()  [unwired: 2 in, 2 out]
        n5390 = property on="MM:" class="DigNum (strict)"("Value"=w6787) -> ()  [unwired: 2 in, 2 out]
        n5391 = property on="HH:" class="DigNum (strict)"("Value"=w6788) -> ()  [unwired: 2 in, 2 out]
        n5392 = property on="Finish Time" class="AbsTime (strict)"("Value"=w6789) -> ()  [unwired: 2 in, 2 out]
      }
      event "Stop Mapping": Value Change {
        n5393 = event-data() -> ()  [unwired: 1 in, 6 out]
        n5394 = Flush Queue(queue=w6819) -> (queue out=w6820:refnum<queue>)  [unwired: 1 in, 2 out]
        n5395 = Enqueue Element(queue=w6820, element="Idle") -> ()  [unwired: 2 in, 3 out]
        n5396 = property on="Start Mapping" class="Bool"("DisabledEnum"=T12."Enabled" ("Disabled")) -> ()  [unwired: 2 in, 2 out]
        n5397 = property on="Stop Mapping" class="Bool"("DisabledEnum"=T12."Disabled and Grayed Out" ("Disabled")) -> ()  [unwired: 2 in, 2 out]
      }
      event "Stop HyperLoop": Value Change {
        n5398 = event-data() -> ()  [unwired: 1 in, 6 out]
        n5399 = Flush Queue(queue=w6824) -> (queue out=w6825:refnum<queue>)  [unwired: 1 in, 2 out]
        n5400 = Enqueue Element(queue=w6825, element="Idle") -> ()  [unwired: 2 in, 3 out]
        n5401 = property on="Start HyperLoop" class="Bool"("DisabledEnum"=T12."Enabled" ("Disabled")) -> ()  [unwired: 2 in, 2 out]
        n5402 = property on="Stop HyperLoop" class="Bool"("DisabledEnum"=T12."Disabled and Grayed Out" ("Disabled")) -> ()  [unwired: 2 in, 2 out]
      }
      event "Stop SuperHyper": Value Change {
        n5403 = event-data() -> ()  [unwired: 1 in, 6 out]
        n5404 = Flush Queue(queue=w6829) -> (queue out=w6830:refnum<queue>)  [unwired: 1 in, 2 out]
        n5405 = Enqueue Element(queue=w6830, element="Idle") -> ()  [unwired: 2 in, 3 out]
        n5406 = property on="StartSuperHyper" class="Bool"("DisabledEnum"=T12."Enabled" ("Disabled")) -> ()  [unwired: 2 in, 2 out]
        n5407 = property on="Stop SuperHyper" class="Bool"("DisabledEnum"=T12."Disabled and Grayed Out" ("Disabled")) -> ()  [unwired: 2 in, 2 out]
      }
      event "Sweep Down": Value Change {
        n5408 = event-data() -> ()  [unwired: 1 in, 6 out]
        n5409 = stacked-sequence {
          tunnel: w6832 -> [_ w6837]
          frame #0 {
            n5410 = property on="Down Rate" class="DigNum (strict)"() -> ("Value"=w6833:dbl)  [unwired: 2 in, 2 out]
            n5411 = property on="lower limit" class="DigNum (strict)"() -> ("Value"=w6834:dbl)  [unwired: 2 in, 2 out]
            n5412 = property on="sweep rate, /min" class="DigNum (strict)"("Value"=w6833) -> ()  [unwired: 2 in, 2 out]
            n5413 = property on="sweep to:" class="DigNum (strict)"("Value"=w6834) -> ()  [unwired: 2 in, 2 out]
            n5414 = property on="Sweep Down" class="Bool"("DisabledEnum"=T12."Disabled and Grayed Out" ("Disabled")) -> ()  [unwired: 2 in, 2 out]
          }
          frame #1 {
            n5415 = Flush Queue(queue=w6837) -> (queue out=w6836:refnum<queue>)  [unwired: 1 in, 2 out]
            n5416 = Enqueue Element(queue=w6836, element="Start Sweep") -> ()  [unwired: 2 in, 3 out]
          }
        }
      }
      event "Sweep Up": Value Change {
        n5417 = event-data() -> ()  [unwired: 1 in, 6 out]
        n5418 = stacked-sequence {
          tunnel: w6839 -> [_ w6844]
          frame #0 {
            w6840 = T12."Disabled and Grayed Out" ("Disabled")
            n5419 = property on="Up Rate" class="DigNum (strict)"() -> ("Value"=w6841:dbl)  [unwired: 2 in, 2 out]
            n5420 = property on="upper limit" class="DigNum (strict)"() -> ("Value"=w6842:dbl)  [unwired: 2 in, 2 out]
            n5421 = property on="sweep rate, /min" class="DigNum (strict)"("Value"=w6841) -> ()  [unwired: 2 in, 2 out]
            n5422 = property on="sweep to:" class="DigNum (strict)"("Value"=w6842) -> ()  [unwired: 2 in, 2 out]
            n5423 = property on="Sweep Down" class="Bool"("DisabledEnum"=w6840) -> ()  [unwired: 2 in, 2 out]
            n5424 = property on="Sweep Up" class="Bool"("DisabledEnum"=w6840) -> ()  [unwired: 2 in, 2 out]
          }
          frame #1 {
            n5425 = Flush Queue(queue=w6844) -> (queue out=w6843:refnum<queue>)  [unwired: 1 in, 2 out]
            n5426 = Enqueue Element(queue=w6843, element="Start Sweep") -> ()  [unwired: 2 in, 3 out]
          }
        }
      }
      event "Ramp\n Down": Value Change {
        n5427 = event-data() -> ()  [unwired: 1 in, 6 out]
        n5428 = Flush Queue(queue=w6847) -> (queue out=w6846:refnum<queue>)  [unwired: 1 in, 2 out]
        n5429 = property on="lower limit" class="DigNum (strict)"() -> ("Value"=w6850:dbl)  [unwired: 2 in, 2 out]
        n5430 = property on="Down Rate" class="DigNum (strict)"() -> ("Value"=w6849:dbl)  [unwired: 2 in, 2 out]
        n5431 = Enqueue Element(queue=w6846, element="Ramp To Limit") -> ()  [unwired: 2 in, 3 out]
        n5432 = property on="sweep to:" class="DigNum (strict)"("Value"=w6850) -> ()  [unwired: 2 in, 2 out]
        n5433 = property on="sweep rate, /min" class="DigNum (strict)"("Value"=w6849) -> ()  [unwired: 2 in, 2 out]
      }
      event "Ramp \nUp": Value Change {
        n5434 = event-data() -> ()  [unwired: 1 in, 6 out]
        n5435 = Flush Queue(queue=w6852) -> (queue out=w6851:refnum<queue>)  [unwired: 1 in, 2 out]
        n5436 = property on="Up Rate" class="DigNum (strict)"() -> ("Value"=w6853:dbl)  [unwired: 2 in, 2 out]
        n5437 = property on="upper limit" class="DigNum (strict)"() -> ("Value"=w6854:dbl)  [unwired: 2 in, 2 out]
        n5438 = Enqueue Element(queue=w6851, element="Ramp To Limit") -> ()  [unwired: 2 in, 3 out]
        n5439 = property on="sweep rate, /min" class="DigNum (strict)"("Value"=w6853) -> ()  [unwired: 2 in, 2 out]
        n5440 = property on="sweep to:" class="DigNum (strict)"("Value"=w6854) -> ()  [unwired: 2 in, 2 out]
      }
      event "Start Mapping", "HyperLoop Hidden": Value Change {
        n5441 = event-data() -> ()  [unwired: 1 in, 6 out]
        n5442 = stacked-sequence {
          tunnel: w6856 -> [_ _ _ _ w6943]
          frame #0 {
            n5443 = property on="Change Sweep Range" class="Bool (strict)"() -> ("Value"=w6857:bool)  [unwired: 2 in, 2 out]
            n5444 = case shown="True" w6857 {
              frame False {
              }
              frame True {
                n5445 = property on="Down          Up" class="Tbl (strict)"("Active Cell"=cluster{"Row":i32, "Column":i32} {"Row"=-2, "Column"=-2}, "Cell BG Color"=u32 16448250 ("Active Cell:Cell Background Color")) -> ()  [unwired: 2 in, 2 out]
              }
            }
            n5446 = property on="Step values" class="Tbl (strict)"("Active Cell"=cluster{"Row":i32, "Column":i32} {"Row"=-2, "Column"=-2}, "Cell BG Color"=u32 16448250 ("Active Cell:Cell Background Color")) -> ()  [unwired: 2 in, 2 out]
          }
          frame #1 {
            # "If change sweep range for different step value, set the sweep range"
            n5447 = property on="Change Sweep Range" class="Bool (strict)"() -> ("Value"=w6862:bool)  [unwired: 2 in, 2 out]
            n5448 = case shown="True" w6862 {
              frame False {
              }
              frame True {
                w6866 = 0 ("disabled index (col)")
                n5449 = property on="Down          Up" class="Tbl (strict)"() -> ("Value"=w6867:string[][])  [unwired: 2 in, 2 out]
                n5450 = Index Array(array=w6867, index (row)=w6866, index (col)=w6866) -> (element=w6868:string)
                n5451 = Index Array(array=w6867, index (row)=w6866, index (col)=1 ("disabled index (col)")) -> (element=w6864:string)
                n5452 = Fract/Exp String To Number(string=w6868) -> (number=w6869:dbl)  [unwired: 3 in, 1 out]
                n5453 = Fract/Exp String To Number(string=w6864) -> (number=w6863:dbl)  [unwired: 3 in, 1 out]
                n5454 = property on="lower limit" class="DigNum (strict)"("Value"=w6869) -> ()  [unwired: 2 in, 2 out]
                n5455 = property on="upper limit" class="DigNum (strict)"("Value"=w6863) -> ()  [unwired: 2 in, 2 out]
              }
            }
          }
          frame #2 {
            n5456 = property on="lower limit" class="DigNum (strict)" props=["Value"]() -> ()  [unwired: 2 in, 3 out]
            n5457 = property on="Stop Mapping" class="Bool"("DisabledEnum"=T12."Enabled" ("Disabled")) -> ()  [unwired: 2 in, 2 out]
            n5458 = property on="upper limit" class="DigNum (strict)"() -> ("Value"=w6870:dbl)  [unwired: 2 in, 2 out]
            n5459 = property on="Down Rate" class="DigNum (strict)"() -> ("Value"=w6873:dbl)  [unwired: 2 in, 2 out]
            n5460 = property on="sweep to:" class="DigNum (strict)"("Value"=w6870) -> ()  [unwired: 2 in, 2 out]
            n5461 = property on="sweep rate, /min" class="DigNum (strict)"("Value"=w6873) -> ()  [unwired: 2 in, 2 out]
            n5462 = property on="Sweep Direction" class="Str"("Value"="Ramp Down" ("String"), "Text.TextColor"=u32 0 ("Text.Text Colors:Text Color")) -> ()  [unwired: 2 in, 2 out]
            n5463 = property on="Start Mapping" class="Bool"("DisabledEnum"=T12."Disabled and Grayed Out" ("Disabled")) -> ()  [unwired: 2 in, 2 out]
            n5464 = property on="Table Index" class="DigNum (strict)"("Value"=0.0 ("Table Index")) -> ()  [unwired: 2 in, 2 out]
          }
          frame #3 {
            n5465 = property on="HyperLoop" class="Bool (strict)"() -> ("Value"=w6877:bool)  [unwired: 2 in, 2 out]
            n5466 = case shown="False" w6877 {
              frame False {
                # "Reserve two name strings for new mapping data file:\none for up\none for down"
                n5467 = property on="Data Folder" class="Path"() -> ("Value"=w6879:path)  [unwired: 2 in, 2 out]
                n5468 = property on="MappingName" class="Str"() -> ("Value"=w6878:string)  [unwired: 2 in, 2 out]
                n5469 = stacked-sequence {
                  tunnel: w6879 -> [w6885 w6916]
                  tunnel: w6878 -> [w6884 w6915]
                  frame #0 {
                    # "Up mapping"
                    n5470 = property on="HyperLoop" class="Bool (strict)"() -> ("Value"=w6881:bool)  [unwired: 2 in, 2 out]
                    n5471 = case shown="False" w6881 {
                      tunnel: ["_up" w6896] -> w6880
                      frame False {
                      }
                      frame True {
                        n5472 = property on="step_hyper" class="RadioBtnsControl (strict)"() -> ("Value"=w6897:T9)  [unwired: 2 in, 2 out]
                        n5473 = case shown="\"iTC_HyperLoop\"" w6897 {
                          tunnel: ["_V2400=" ("string") "_V2400=" ("string") "_Va=" ("string") "_Vb=" ("string") "_t=" ("string") "_T=" ("string") "_B" ("string")] -> w6892
                          tunnel: ["V" ("string") "V" ("string") "V" ("string") "V" ("string") _ "K" ("string") "T" ("string")] -> w6891
                          frame "2400_1_HyperLoop", Default {
                          }
                          frame "2400_2_HyperLoop" {
                          }
                          frame "2636_smua_HyperLoop" {
                          }
                          frame "2636_smub_HyperLoop" {
                          }
                          frame "time_HyperLoop" {
                          }
                          frame "iTC_HyperLoop" {
                          }
                          frame "iPS_HyperLoop" {
                          }
                        }
                        n5474 = property on="Current Hyper Value" class="DigNum (strict)"() -> ("Value"=w6894:dbl)  [unwired: 2 in, 2 out]
                        n5475 = Number To Exponential String(number=w6894) -> (E-format string=w6893:string)  [unwired: 3 in]
                        n5476 = Concatenate Strings("_up" ("string"), w6892, w6893, w6891) -> (w6896:string)
                      }
                    }
                    n5477 = Concatenate Strings(w6884, w6880) -> (w6882:string)
                    n5478 = call "AutoNamerDatExtraArtem.vi"("SweepType"=w6882, "Custom User Path"=w6885) -> ("String"=w6888:string, "Path"=w6889:path)  [unwired: 2 in]
                    n5479 = Path To String(path=w6889) -> (string=w6887:string)
                    n5480 = Concatenate Strings(w6887, "\\", w6888) -> (→"UpNameString":string)
                  }
                  frame #1 {
                    # "Down mapping"
